vi "SAVE_PATH.vi"(7 "chn_in":i32, 8 "Sampling":bool, 9 "Temperature":bool, 10 "filename":string, 11 "folder":path) -> (0 "path":path, 1 "Newfile":bool, 2 "save_filename":string, 3 "Channel":string, 4 "filename_for_cfg":string)   [LabVIEW 2015]
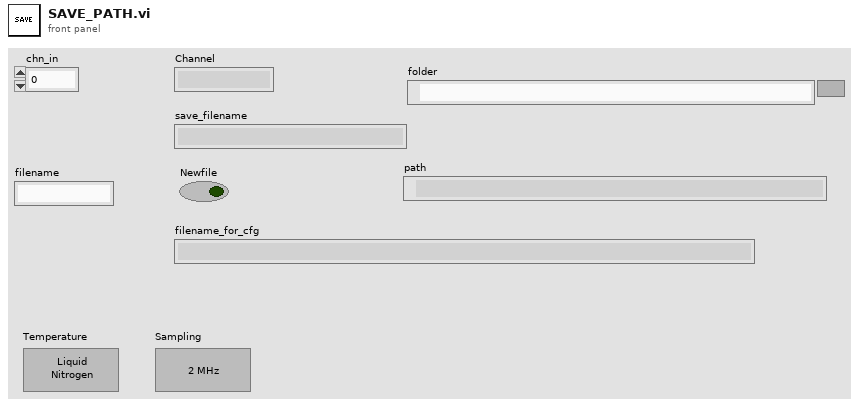
[diagram p1: front panel]
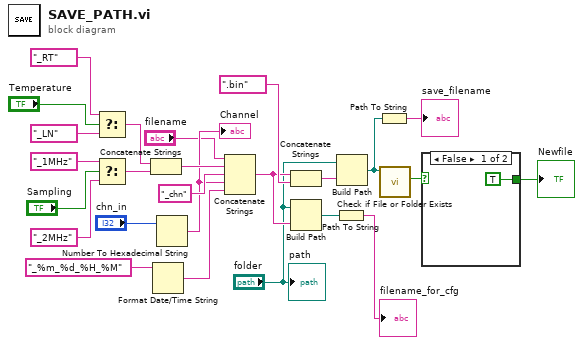
[diagram p0: block diagram]
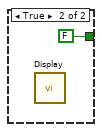
[diagram p2: hidden frame]
diagram:
  n1 = Select(t="_RT" ("string"), s="Temperature", f="_LN" ("string")) -> (s? t:f=w10:string)
  n2 = Select(t="_1MHz" ("string"), s="Sampling", f="_2MHz" ("string")) -> (s? t:f=w9:string)
  n3 = Concatenate Strings(w10, w9) -> (w8:string)
  n4 = Format Date/Time String(time format string (%c)="_%m_%d_%H_%M") -> (date/time string=w22:string)  [unwired: 2 in]
  n5 = Number To Hexadecimal String(2:"chn_in") -> (0:w6:string)  [unwired: 1 in]
  "Channel" <- w6
  n6 = Concatenate Strings("filename", w8, "_chn" ("string"), w6, w22) -> (w5:string)
  n7 = Concatenate Strings(w5, ".bin" ("string")) -> (w25:string)
  n8 = Build Path(base path="folder", name or relative path=w5) -> (appended path=w4:path)
  n9 = Path To String(path=w4) -> (string=→"filename_for_cfg":string)
  n10 = Build Path(base path="folder", name or relative path=w25) -> (appended path=w18:path)
  n11 = Path To String(path=w18) -> (string=→"save_filename":string)
  n12 = call <vilib>:"Check if File or Folder Exists.vi"("path"=w18) -> ("file or folder exists?"=w19:bool)  [unwired: 8 in, 2 out]
  n13 = case shown="False" w19 {
    tunnel: [TRUE ("T button?") FALSE ("T button?")] -> w23
    frame False {
    }
    frame True {
      n14 = call "Display"() -> ()  [unwired: 10 in, 2 out]
    }
  }
  "Newfile" <- w23
  "path" <- "folder"
